vi "CoffeeMachine.vi"(11 "error in":errorcluster) -> (15 "error out":errorcluster)   [LabVIEW 2020]
uses:
  TypeDefs/QueueOperations.ctl
  TypeDefs/DataCluster.ctl
  <vilib>/Utility/config.llb/Read Key (Boolean).vi
  <vilib>/Utility/config.llb/Read Key (I32).vi
  <vilib>/Utility/config.llb/NI_LVConfig.lvlib
panel:
  out "Total Cups":i32
  out "ElapsedTime":dbl
  in  "Power":bool
  out "Brewing":bool
  out "Grinding":bool
  out "Heating":bool
  out "Dispensing":bool
  out "Purging":bool
  out "Dispenser":dbl(slide) scale=0.0..10.0
  out "Chamber":dbl(slide) scale=0.0..10.0
  out "Low Milk":bool
  out "Low Bean":bool
  out "Low Water":bool
  in  "Milk Level":dbl(slide) scale=0.0..100.0
  in  "Bean Level":dbl(slide) scale=0.0..100.0
  in  "Carafe":bool
  in  "Cup":bool
  in  "UserChoice":i32(knob) scale=0.0..2.0
  in  "Water Level":dbl(slide) scale=0.0..100.0
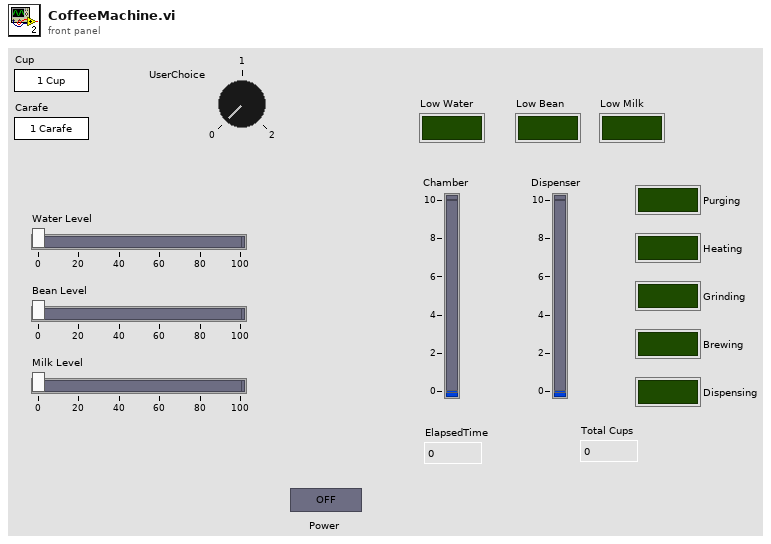
[diagram p1: front panel]
types:
  T1 = typedef "DataCluster.ctl" = cluster{"Dispenser":dbl, "Chamber":dbl, "Low Water":bool, "Low Bean":bool, "Low Milk":bool, "Purging":bool, "Dispensing":bool, "Heating":bool, "Grinding":bool, "Brewing":bool, "UserChoice":i32, "Power":bool, "Water Level":dbl, "Carafe":bool, "Cup":bool, "Milk Level":dbl, "Bean Level":dbl, "ProperShutdown?":bool, "PowerTime":dbl[], "PowerSequence":string[], "PowerStartTime":dbl, "ElapsedTime":dbl, "IndexPower":i32, "DoneState":bool, "CupCount":i32, "BeverageTime":dbl[], "BeverageSequence":string[], "BeverageStartTime":dbl, "IndexBeverageSeq":i32, "BeverageTime?":bool, "UserChoiceMade?":bool}
  T2 = typedef "QueueOperations.ctl" = enum16{"Obtain", "Enqueue", "Enstack", "EnqueueArray", "Dequeue", "Flush", "Release"}
  T3 = typedef "NI_LVConfig.lvlib/Config Data RefNum.ctl" = refnum<k1>
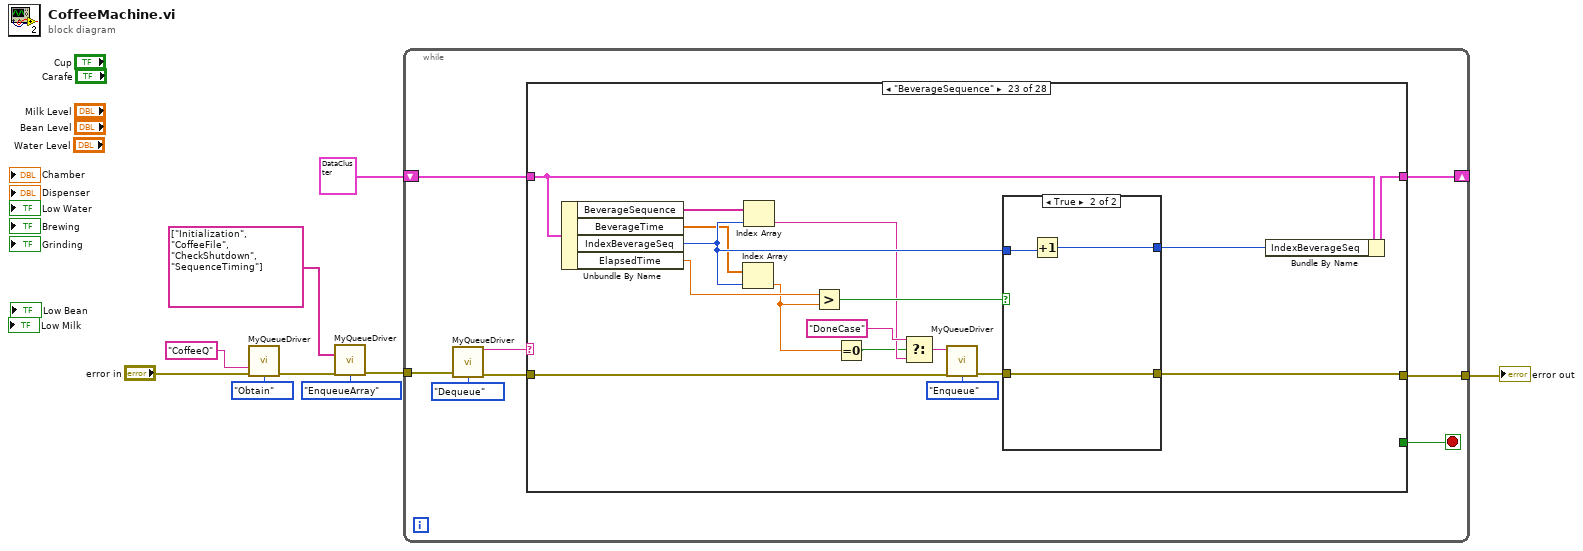
[diagram p0: block diagram]
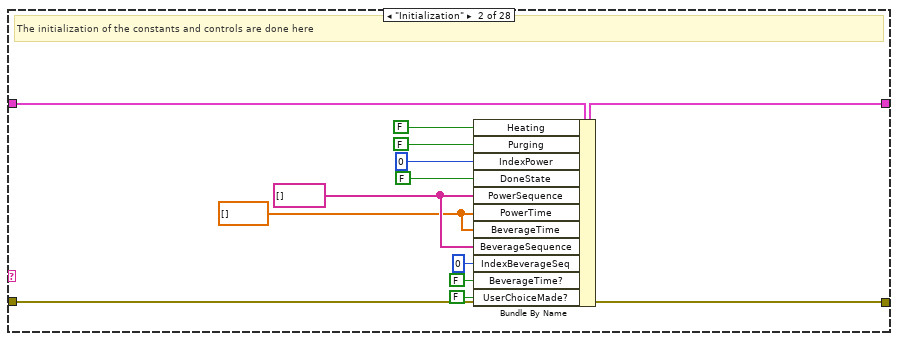
[diagram p3: hidden frame]
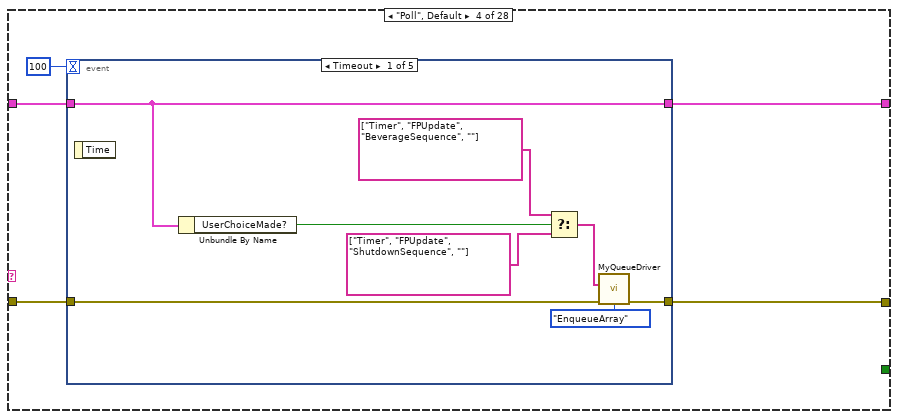
[diagram p5: hidden frame]
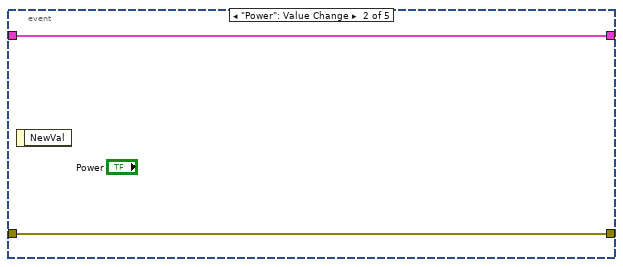
[diagram p6: hidden frame]
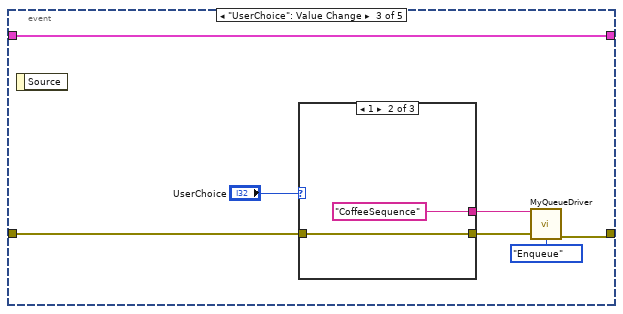
[diagram p7: hidden frame]
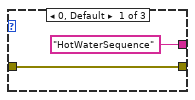
[diagram p8: hidden frame]
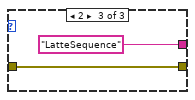
[diagram p9: hidden frame]
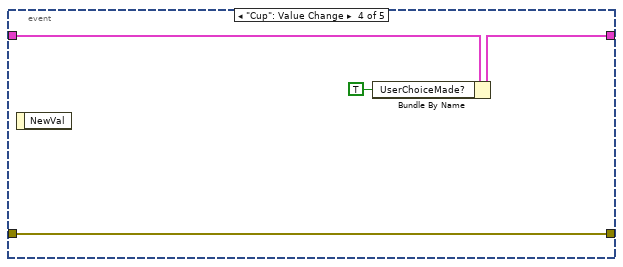
[diagram p10: hidden frame]
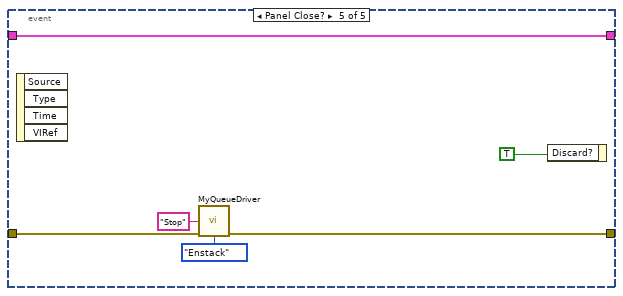
[diagram p11: hidden frame]
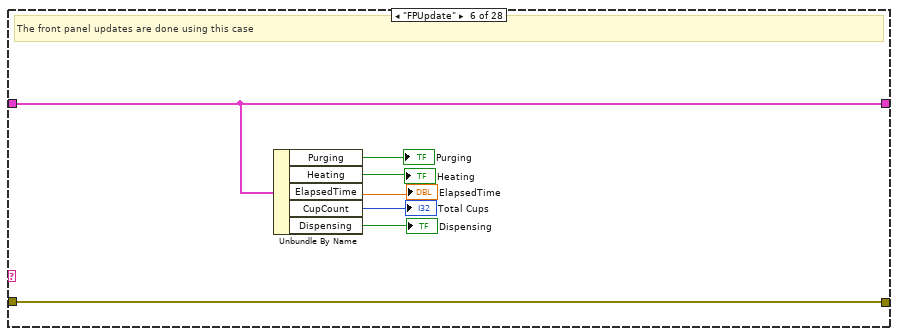
[diagram p13: hidden frame]
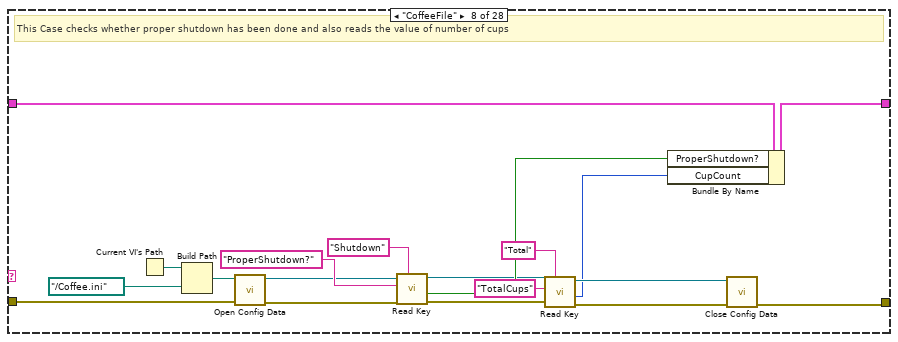
[diagram p15: hidden frame]
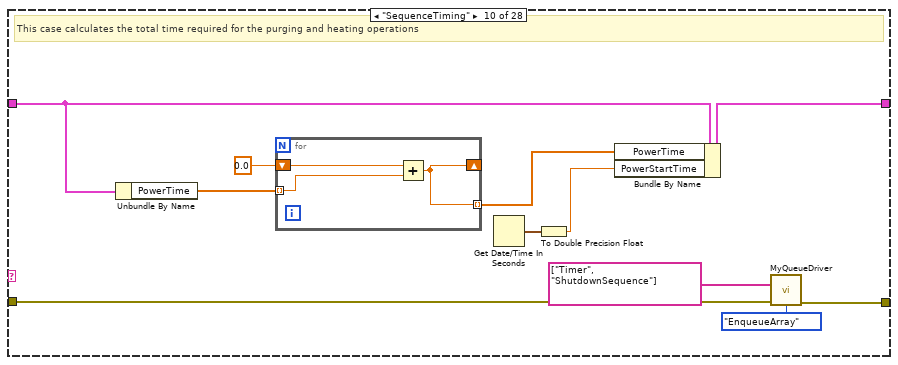
[diagram p17: hidden frame]
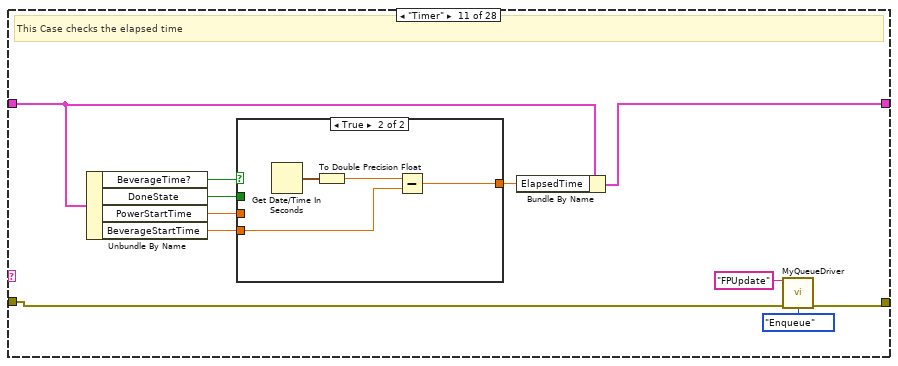
[diagram p18: hidden frame]
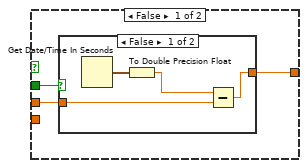
[diagram p19: hidden frame]
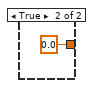
[diagram p20: hidden frame]
diagram:
  n1 = call "MyQueueDriver.vi"("name"="CoffeeQ", "error in"="error in", "Operation"=QueueOperations."Obtain") -> ("error out"=w6:errorcluster)  [unwired: 11 in, 1 out]
  n2 = call "MyQueueDriver.vi"("StateArray"=string[] ["Initialization", "CoffeeFile", "CheckShutdown", "SequenceTiming"], "error in"=w6, "Operation"=QueueOperations."EnqueueArray") -> ("error out"=w3:errorcluster)  [unwired: 11 in, 1 out]
  n3 = while {
    tunnel: w3 -> [w16]
    shift-right: [w12] -> _
    shift-left: T1 {"Dispenser"=0.0, "Chamber"=0.0, "Low Water"=FALSE, "Low Bean"=FALSE, "Low Milk"=FALSE, "Purging"=FALSE, "Dispensing"=FALSE, "Heating"=FALSE, "Grinding"=FALSE, "Brewing"=FALSE, "UserChoice"=0, "Power"=FALSE, "Water Level"=0.0, "Carafe"=FALSE, "Cup"=FALSE, "Milk Level"=0.0, "Bean Level"=0.0, "ProperShutdown?"=FALSE, "PowerTime"=[], "PowerSequence"=[], "PowerStartTime"=0.0, "ElapsedTime"=0.0, "IndexPower"=0, "DoneState"=FALSE, "CupCount"=0, "BeverageTime"=[], "BeverageSequence"=[], "BeverageStartTime"=0.0, "IndexBeverageSeq"=0, "BeverageTime?"=FALSE, "UserChoiceMade?"=FALSE} -> [w13]
    tunnel: [w11] -> w1
    stop <- w10 stop-if-true
    n4 = call "MyQueueDriver.vi"("error in"=w16, "Operation"=QueueOperations."Dequeue") -> ("Dequeued Element"=w14:string, "error out"=w15:errorcluster)  [unwired: 12 in]
    n5 = case shown="\"BeverageSequence\"" w14 {
      tunnel: w15 -> [w18 w31 w32 w36 w72 w77 w81 w101 w102 w105 w123 w141 w144 w167 w182 w187 w192 w197 w202 w213 w219 w228 w242 w256 w263 w269 w272 w279]
      tunnel: w13 -> [w19 w30 w33 w37 w73 w80 w82 w94 w103 w112 w127 w142 w146 w170 w184 w191 w194 w198 w207 w209 w215 w222 w232 w262 w264 w265 w273 w280]
      tunnel: [w19 w27 w33 w34 w73 w80 w82 w93 w103 w110 w128 w142 w145 w164 w183 w190 w193 w198 w206 w208 w214 w221 w239 w261 w264 w265 w273 w280] -> w12
      tunnel: [w18 w31 w32 w35 w72 w77 w81 w84 w102 w104 w122 w141 w143 w165 w182 w187 w192 w197 w201 w213 w219 w228 w240 w255 w263 w267 w272 w275] -> w11
      tunnel: [_ _ _ _ _ _ _ _ _ _ _ _ _ _ _ _ _ _ _ _ _ _ _ _ _ TRUE _ _] -> w10
      frame "-----Initialization-----" {
      }
      frame "Initialization" {
        w23 = dbl[] [] ("PowerTime")
        w24 = string[] [] ("PowerSequence")
        # "The initialization of the constants and controls are done here"
        n6 = Bundle By Name(cluster=w30, "Heating"=FALSE, "Purging"=FALSE, "IndexPower"=0 ("IndexShiftRegister"), "DoneState"=FALSE, "PowerSequence"=w24, "PowerTime"=w23, "BeverageTime"=w23, "BeverageSequence"=w24, "IndexBeverageSeq"=0, "BeverageTime?"=FALSE, "UserChoiceMade?"=FALSE) -> (w27:T1)
      }
      frame "-----Poll-----" {
      }
      frame "Poll", Default {
        n7 = event shown="[0] Timeout" {
          selector: _ -> [_ _ _ _ _]
          dyn-events: _ -> [_ _ _ _ _]
          timeout: 100 -> [_ _ _ _ _]
          tunnel: w37 -> [w43 w48 w50 w65 w66]
          tunnel: w36 -> [w45 w47 w54 w62 w70]
          tunnel: [w44 w47 w51 w62 w69] -> w35
          tunnel: [w43 w48 w50 w64 w66] -> w34
          event Timeout {
            n8 = event-data() -> ()  [unwired: 1 in, 1 out]
            n9 = Unbundle By Name(w43) -> ("UserChoiceMade?"=w40:bool)
            n10 = Select(t=string[] ["Timer", "FPUpdate", "BeverageSequence", ""] ("StateArray"), s=w40, f=string[] ["Timer", "FPUpdate", "ShutdownSequence", ""] ("StateArray")) -> (s? t:f=w39:string[])
            n11 = call "MyQueueDriver.vi"("StateArray"=w39, "error in"=w45, "Operation"=QueueOperations."EnqueueArray") -> ("error out"=w44:errorcluster)  [unwired: 11 in, 1 out]
          }
          event "Power": Value Change {
            n12 = event-data() -> ()  [unwired: 1 in, 1 out]
          }
          event "UserChoice": Value Change {
            n13 = event-data() -> ()  [unwired: 1 in, 1 out]
            n14 = case shown="1" "UserChoice" {
              tunnel: w54 -> [w57 w59 w61]
              tunnel: [w57 w59 w61] -> w52
              tunnel: ["HotWaterSequence" ("Element To Enqueue") "CoffeeSequence" ("Element To Enqueue") "LatteSequence" ("Element To Enqueue")] -> w49
              frame 0, Default {
              }
              frame 1 {
              }
              frame 2 {
              }
            }
            n15 = call "MyQueueDriver.vi"("Element To Enqueue"=w49, "error in"=w52, "Operation"=QueueOperations."Enqueue") -> ("error out"=w51:errorcluster)  [unwired: 11 in, 1 out]
          }
          event "Cup": Value Change {
            n16 = event-data() -> ()  [unwired: 1 in, 1 out]
            n17 = Bundle By Name(cluster=w65, "UserChoiceMade?"=TRUE) -> (w64:T1)
          }
          event Panel Close? {
            n18 = event-data() -> ()  [unwired: 1 in, 4 out]
            n19 = call "MyQueueDriver.vi"("Element To Enstack"="Stop", "error in"=w70, "Operation"=QueueOperations."Enstack") -> ("error out"=w69:errorcluster)  [unwired: 11 in, 1 out]
            n20 = event-data("Discard?"=TRUE) -> ()  [unwired: 1 in, 1 out]
          }
        }
      }
      frame "-----FPUpdate-----" {
      }
      frame "FPUpdate" {
        # "The front panel updates are done using this case"
        n21 = Unbundle By Name(w80) -> ("Purging"=→"Purging":bool, "Heating"=→"Heating":bool, "ElapsedTime"=→"ElapsedTime":dbl, "CupCount"=→"Total Cups":i32, "Dispensing"=→"Dispensing":bool)
      }
      frame "-----FileData-----" {
      }
      frame "CoffeeFile" {
        # "This Case checks whether proper shutdown has been done and also reads the value of number of cups"
        n22 = Current VI's Path() -> (path=w100:path)
        n23 = Build Path(base path=w100, name or relative path=path "../Coffee.ini") -> (appended path=w98:path)
        n24 = call <vilib>:"Open Config Data.vi"("error in (no error)"=w101, "configuration file path"=w98) -> ("error out"=w97:errorcluster, "refnum"=w91:T3)  [unwired: 7 in, 1 out]
        n25 = call-poly <vilib>:"Read Key.vi"("section"="Shutdown", "error in (no error)"=w97, "key"="ProperShutdown?", "refnum"=w91) -> ("error out"=w90:errorcluster, "value"=w92:bool, "refnum out"=w86:T3)  [unwired: 4 in, 1 out]
        n26 = call-poly <vilib>:"Read Key.vi"("section"="Total", "error in (no error)"=w90, "key"="TotalCups", "refnum"=w86) -> ("error out"=w87:errorcluster, "value"=w83:i32, "refnum out"=w85:T3)  [unwired: 4 in, 1 out]
        n27 = Bundle By Name(cluster=w94, "ProperShutdown?"=w92, "CupCount"=w83) -> (w93:T1)
        n28 = call <vilib>:"Close Config Data.vi"("error in (no error)"=w87, "refnum"=w85) -> ("error out"=w84:errorcluster)  [unwired: 8 in, 1 out]
      }
      frame "-----Timer-----" {
      }
      frame "SequenceTiming" {
        # "This case calculates the total time required for the purging and heating operations"
        n29 = Unbundle By Name(w112) -> ("PowerTime"=w114:dbl[])
        n30 = for {
          tunnel: w114 -> [w116] mode=indexing
          shift-right: [w115] -> _
          shift-left: 0.0 -> [w117]
          tunnel: [w115] -> w111 mode=indexing
          n31 = Add(x=w117, y=w116) -> (x+y=w115:dbl)
        }
        n32 = Get Date/Time In Seconds() -> (seconds since 1Jan1904=w109:timestamp)
        n33 = To Double Precision Float(number=w109) -> (double precision float=w108:dbl)
        n34 = Bundle By Name(cluster=w112, "PowerTime"=w111, "PowerStartTime"=w108) -> (w110:T1)
        n35 = call "MyQueueDriver.vi"("StateArray"=string[] ["Timer", "ShutdownSequence"], "error in"=w105, "Operation"=QueueOperations."EnqueueArray") -> ("error out"=w104:errorcluster)  [unwired: 11 in, 1 out]
      }
      frame "Timer" {
        # "This Case checks the elapsed time"
        n36 = Unbundle By Name(w127) -> ("BeverageTime?"=w119:bool, "DoneState"=w120:bool, "PowerStartTime"=w126:dbl, "BeverageStartTime"=w118:dbl)
        n37 = case shown="True" w119 {
          tunnel: w126 -> [w131 _]
          tunnel: [w130 w137] -> w125
          tunnel: w120 -> [w129 _]
          tunnel: w118 -> [_ w138]
          frame False {
            n38 = case shown="False" w129 {
              tunnel: w131 -> [w133 _]
              tunnel: [w132 0.0] -> w130
              frame False {
                n39 = Get Date/Time In Seconds() -> (seconds since 1Jan1904=w135:timestamp)
                n40 = To Double Precision Float(number=w135) -> (double precision float=w134:dbl)
                n41 = Subtract(x=w134, y=w133) -> (x-y=w132:dbl)
              }
              frame True {
              }
            }
          }
          frame True {
            n42 = Get Date/Time In Seconds() -> (seconds since 1Jan1904=w140:timestamp)
            n43 = To Double Precision Float(number=w140) -> (double precision float=w139:dbl)
            n44 = Subtract(x=w139, y=w138) -> (x-y=w137:dbl)
          }
        }
        n45 = Bundle By Name(cluster=w127, "ElapsedTime"=w125) -> (w128:T1)
        n46 = call "MyQueueDriver.vi"("Element To Enqueue"="FPUpdate", "error in"=w123, "Operation"=QueueOperations."Enqueue") -> ("error out"=w122:errorcluster)  [unwired: 11 in, 1 out]
      }
      frame "-----PowerSequence-----" {
      }
      frame "CheckShutdown" {
        n47 = Unbundle By Name(w146) -> ("ProperShutdown?"=w147:bool)
        n48 = case shown="False" w147 {
          tunnel: w146 -> [w151 w154]
          tunnel: [w150 w153] -> w145
          tunnel: w144 -> [w152 w157]
          tunnel: [w152 w157] -> w143
          frame False {
            n49 = Bundle By Name(cluster=w151, "PowerTime"=dbl[] [4.0, 5.0], "PowerSequence"=string[] ["Purging", "Heating"]) -> (w150:T1)
          }
          frame True {
            n50 = Bundle By Name(cluster=w154, "PowerTime"=dbl[] [5.0, 0.0], "PowerSequence"=string[] ["Heating", ""]) -> (w153:T1)
          }
        }
      }
      frame "ShutdownSequence" {
        n51 = Unbundle By Name(w170) -> ("PowerSequence"=w174:string[], "PowerTime"=w163:dbl[], "IndexPower"=w171:i32, "ElapsedTime"=w173:dbl)
        n52 = Index Array(array=w163, index=w171) -> (element=w158:dbl)
        n53 = Index Array(array=w174, index=w171) -> (element=w161:string)
        n54 = Greater?(x=w173, y=w158) -> (0:w172:bool)
        n55 = Equal To 0?(x=w158) -> (x = 0?=w159:bool)
        n56 = Select(t="DoneCase" ("element"), s=w159, f=w161) -> (s? t:f=w160:string)
        n57 = call "MyQueueDriver.vi"("Element To Enqueue"=w160, "error in"=w167, "Operation"=QueueOperations."Enqueue") -> ("error out"=w166:errorcluster)  [unwired: 11 in, 1 out]
        n58 = case shown="False" w172 {
          tunnel: w171 -> [w176 w179]
          tunnel: [w176 w178] -> w169
          tunnel: w166 -> [w175 w177]
          tunnel: [w175 w177] -> w165
          frame False {
          }
          frame True {
            n59 = Increment(x=w179) -> (x+1=w178:i32)
          }
        }
        n60 = Bundle By Name(cluster=w170, "IndexPower"=w169) -> (w164:T1)
      }
      frame "DoneCase" {
        n61 = Bundle By Name(cluster=w184, "Heating"=FALSE, "Purging"=FALSE, "DoneState"=TRUE, "Dispensing"=FALSE) -> (w183:T1)
      }
      frame "Heating" {
        n62 = Bundle By Name(cluster=w191, "Heating"=TRUE, "Purging"=FALSE) -> (w190:T1)
      }
      frame "Purging" {
        n63 = Bundle By Name(cluster=w194, "Heating"=FALSE, "Purging"=TRUE) -> (w193:T1)
      }
      frame "-----BeverageSequence-----" {
      }
      frame "HotWaterSequence" {
        n64 = call "MyQueueDriver.vi"("StateArray"=string[] ["BeverageStartTime", "Timer", "BeverageSequence"], "error in"=w202, "Operation"=QueueOperations."EnqueueArray") -> ("error out"=w201:errorcluster)  [unwired: 11 in, 1 out]
        n65 = Bundle By Name(cluster=w207, "BeverageTime"=dbl[] [5.0], "BeverageSequence"=string[] ["Dispensing"], "DoneState"=FALSE) -> (w206:T1)
      }
      frame "CoffeeSequence" {
        n66 = Bundle By Name(cluster=w209, "BeverageTime"=dbl[] [3.0, 4.0, 5.0], "BeverageSequence"=string[] ["Grinding", "Brewing", "Dispensing", ""], "DoneState"=FALSE) -> (w208:T1)
      }
      frame "LatteSequence" {
        n67 = Bundle By Name(cluster=w215, "BeverageTime"=dbl[] [3.0, 4.0, 5.0], "BeverageSequence"=string[] ["Grinding", "Brewing", "Dispensing"], "DoneState"=FALSE) -> (w214:T1)
      }
      frame "BeverageStartTime" {
        n68 = Unbundle By Name(w222) -> ("BeverageTime"=w227:dbl[])
        n69 = for {
          tunnel: w227 -> [w230] mode=indexing
          shift-right: [w229] -> _
          shift-left: 0.0 -> [w231]
          tunnel: [w229] -> w225 mode=indexing
          n70 = Add(x=w231, y=w230) -> (x+y=w229:dbl)
        }
        n71 = Get Date/Time In Seconds() -> (seconds since 1Jan1904=w224:timestamp)
        n72 = To Double Precision Float(number=w224) -> (double precision float=w223:dbl)
        n73 = Bundle By Name(cluster=w222, "BeverageTime"=w225, "BeverageStartTime"=w223, "BeverageTime?"=TRUE) -> (w221:T1)
      }
      frame "BeverageSequence" {
        n74 = Unbundle By Name(w232) -> ("BeverageSequence"=w248:string[], "BeverageTime"=w238:dbl[], "IndexBeverageSeq"=w245:i32, "ElapsedTime"=w247:dbl)
        n75 = Index Array(array=w238, index=w245) -> (element=w233:dbl)
        n76 = Index Array(array=w248, index=w245) -> (element=w236:string)
        n77 = Greater?(x=w247, y=w233) -> (0:w246:bool)
        n78 = Equal To 0?(x=w233) -> (x = 0?=w234:bool)
        n79 = Select(t="DoneCase" ("element"), s=w234, f=w236) -> (s? t:f=w235:string)
        n80 = call "MyQueueDriver.vi"("Element To Enqueue"=w235, "error in"=w242, "Operation"=QueueOperations."Enqueue") -> ("error out"=w241:errorcluster)  [unwired: 11 in, 1 out]
        n81 = case shown="True" w246 {
          tunnel: w245 -> [w250 w253]
          tunnel: [w250 w252] -> w244
          tunnel: w241 -> [w249 w251]
          tunnel: [w249 w251] -> w240
          frame False {
          }
          frame True {
            n82 = Increment(x=w253) -> (x+1=w252:i32)
          }
        }
        n83 = Bundle By Name(cluster=w232, "IndexBeverageSeq"=w244) -> (w239:T1)
      }
      frame "Dispensing" {
        n84 = call "MyQueueDriver.vi"("Element To Enqueue"="FPUpdate", "error in"=w256, "Operation"=QueueOperations."Enqueue") -> ("error out"=w255:errorcluster)  [unwired: 11 in, 1 out]
        n85 = Bundle By Name(cluster=w262, "Dispensing"=TRUE, "Brewing"=FALSE, "Grinding"=FALSE) -> (w261:T1)
      }
      frame "-----Exit-----" {
      }
      frame "Stop" {
        n86 = call "MyQueueDriver.vi"("error in"=w269, "Operation"=QueueOperations."Flush") -> ("error out"=w268:errorcluster)  [unwired: 12 in, 1 out]
        n87 = call "MyQueueDriver.vi"("error in"=w268, "Operation"=QueueOperations."Release") -> ("error out"=w267:errorcluster)  [unwired: 12 in, 1 out]
      }
      frame "-----Error-----" {
      }
      frame "Error" {
        n88 = Unbundle By Name(w279) -> ("code"=w278:i32, "source"=w277:string)
        n89 = call <vilib>:"Simple Error Handler.vi"("error code (no error:0)"=w278, "error source (\" \")"=w277, "error in (no error)"=w279) -> ("code out"=w274:i32, "error out"=w276:errorcluster)  [unwired: 2 in, 3 out]
        n90 = call <vilib>:"Clear Errors.vi"("error in (no error)"=w276, "specific error code to clear (0: all)"=w274) -> ("error out"=w275:errorcluster)  [unwired: 4 in, 1 out]
      }
    }
  }
  "error out" <- w1
